vi "InitializeNetworkStreamWriter.vi"(11 "Boat Type":T1(ring)) -> (0 "error out":errorcluster, 3 "NetworkStreamWriter out":refnum<class "NetworkStreamWriter.lvclass">)   [LabVIEW 2013]
doc: "Initializes the Writer network stream."
uses:
  RIO-OCU_Comm/NetworkStreams/Writer/NetworkStreamWriter.lvclass
  Location of Think.ctl
  RIO-OCU_Comm/ToRIO.ctl
  CommandMessages.ctl
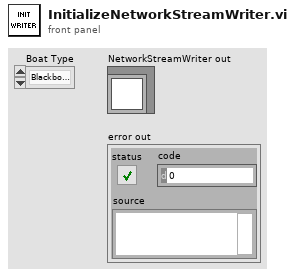
[diagram p1: front panel]
types:
  T1 = enum16{"Blackbody Radiation", "Little boats", "Simulation", "Damn Yankee"}
  T2 = typedef "CommandMessages.ctl" = enum16{"Pass", "OverrideMode", "Add mission", "Delete mission", "Add obstacle", "Delete obstacle", "Change constants"}
  T3 = typedef "ToRIO.ctl" = cluster{"Commands":T2, "Variant":variant}
  T4 = typedef "Location of Think.ctl" = string
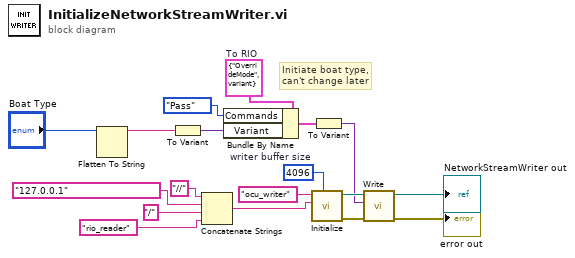
[diagram p0: block diagram]
diagram:
  w7 = T3 {"Commands"=enum."OverrideMode", "Variant"=variant}  # To RIO
  w1 = 4096  # writer buffer size
  # "Initiate boat type,\ncan't change later"
  n1 = Flatten To String(anything="Boat Type") -> (data string=w18:string)  [unwired: 3 in, 2 out]
  n2 = To Variant(anything=w18) -> (Variant=w15:variant)
  n3 = Concatenate Strings("//" ("string"), T4 "127.0.0.1" ("Location of THINK"), "/", "rio_reader" ("string")) -> (w4:string)
  n4 = Bundle By Name(cluster=w7, "Commands"=CommandMessages."Pass", "Variant"=w15) -> (w16:T3)
  n5 = call "Initialize.vi"("writer buffer size"=w1, "reader url"=w4, "writer name"="ocu_writer") -> ("error out"=w11:errorcluster, "NetworkStreamWriter out"=w10:refnum<class "NetworkStreamWriter.lvclass">)  [unwired: 7 in]
  n6 = To Variant(anything=w16) -> (Variant=w8:variant)
  n7 = call "Write.vi"("error in (no error)"=w11, "element"=w8, "NetworkStreamWriter in"=w10) -> ("error out"=→"error out":errorcluster, "NetworkStreamWriter out"=→"NetworkStreamWriter out":refnum<class "NetworkStreamWriter.lvclass">)  [unwired: 7 in]
